vi "parce_string_to_elements.vi"(11 "BSONbytes":u8[](array[numeric]) format="%02x") -> (1 "restOfBytes":u8[](array[numeric]), 2 "sezeOK":bool, 3 "arrayOfElements":T1[](array[typedef]))   [LabVIEW 2015, in "BSON_convertors_Library.lvlib"]
doc: "Created by Artem Shevelev\nLabVIEW Portal profile: http://www.labviewportal.org/memberlist.php?mode=viewprofile&u=2340\ne-mail: artem.sh@gmail.com\nshevelev.pro"
uses:
  BSON_convertors_Library.lvlib
  typedefs/BSONelement.ctl
  typedefs/dataType.ctl
  typedefs/binaryData_cluster.ctl
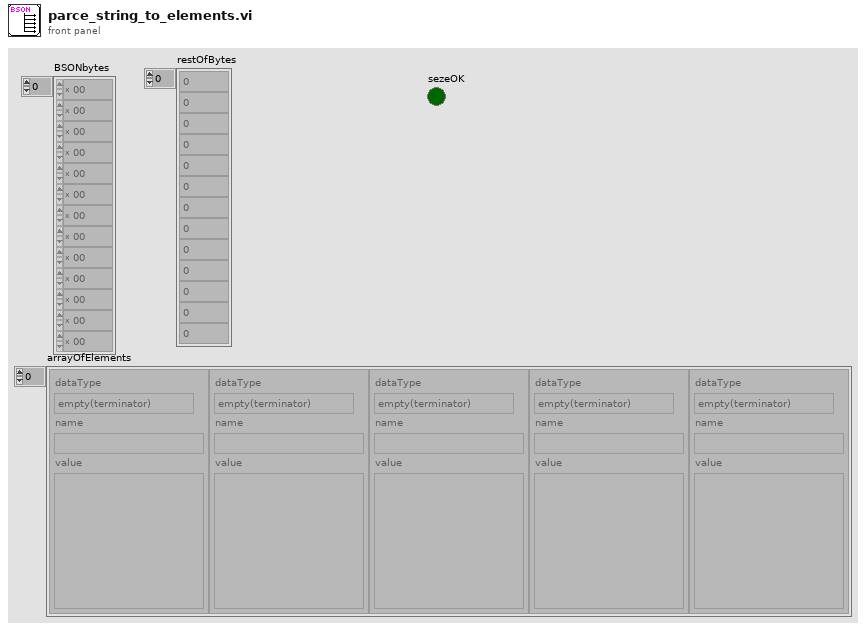
[diagram p1: front panel]
types:
  T1 = typedef "BSON_convertors_Library.lvlib/BSONelement.ctl" = cluster{"dataType":T2, "name":string, "value":variant}
  T2 = typedef "BSON_convertors_Library.lvlib/dataType.ctl" = enum8{"empty(terminator)", "double", "string", "document", "array", "binary", "Deprecated(Undefined)", "ObjectId", "boolean", "UTC datetime", "Null value", "cstring", "Deprecated(DBPointer)", "JavaScript", "Deprecated(Symbol)", "code_w_s", "int32", "uint64", "int64", "ext (decimal128)", "Min key", "Max key"}
  T3 = typedef "BSON_convertors_Library.lvlib/binaryData_cluster.ctl" = cluster{"subType":u8, "byteArray":u8[]}
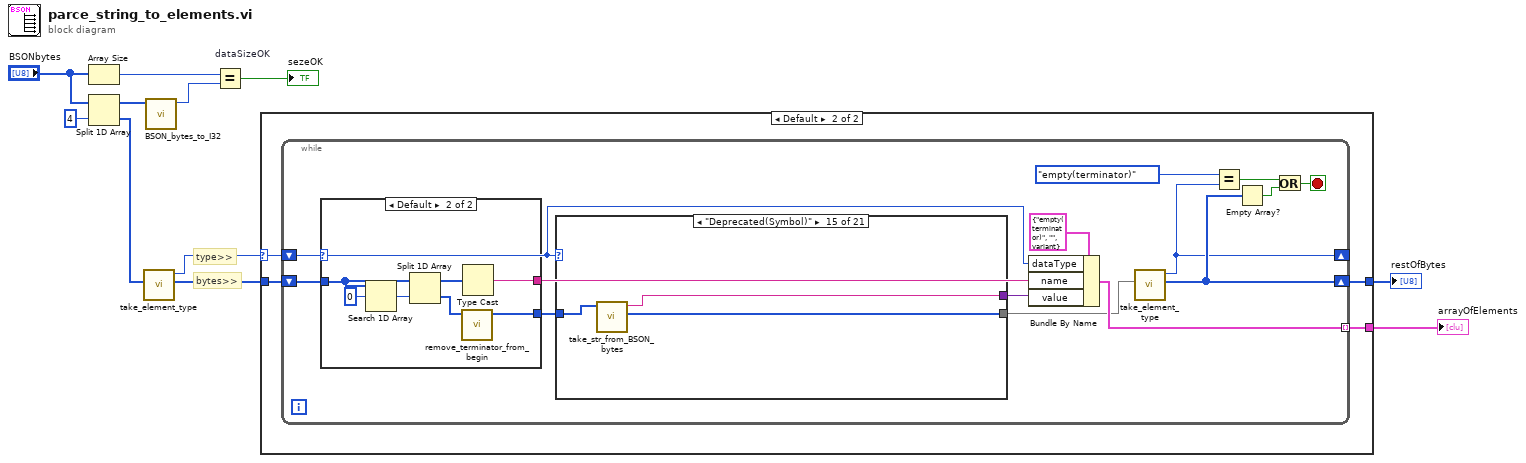
[diagram p0: block diagram]
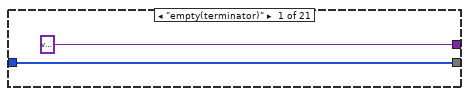
[diagram p4: hidden frame]
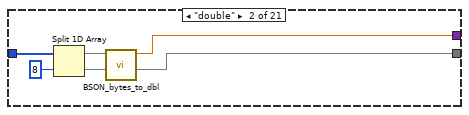
[diagram p5: hidden frame]
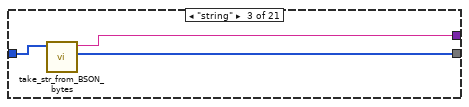
[diagram p6: hidden frame]
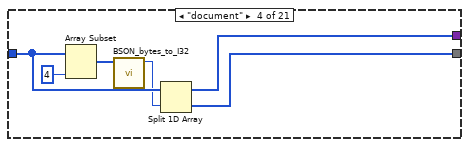
[diagram p7: hidden frame]
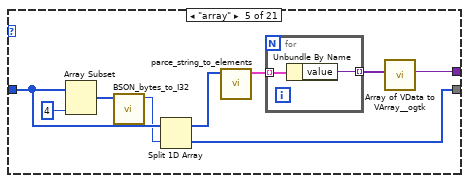
[diagram p8: hidden frame]
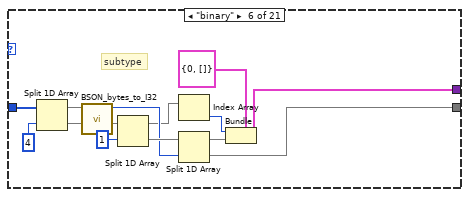
[diagram p9: hidden frame]
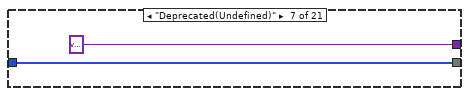
[diagram p10: hidden frame]
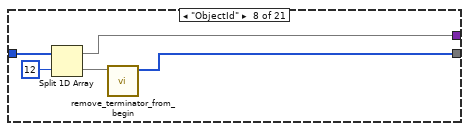
[diagram p11: hidden frame]
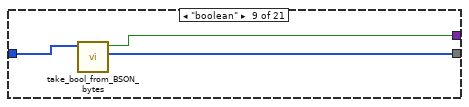
[diagram p12: hidden frame]
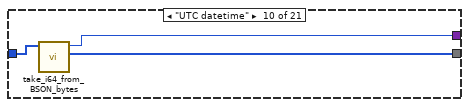
[diagram p13: hidden frame]
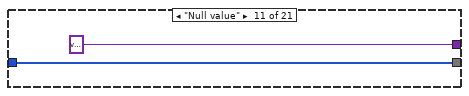
[diagram p14: hidden frame]
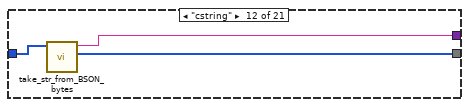
[diagram p15: hidden frame]
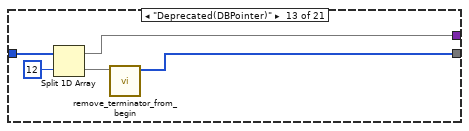
[diagram p16: hidden frame]
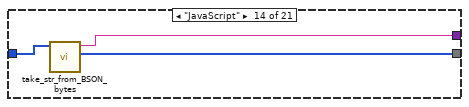
[diagram p17: hidden frame]
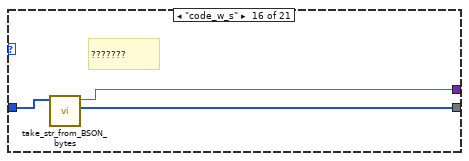
[diagram p18: hidden frame]
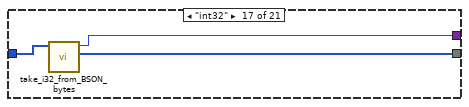
[diagram p19: hidden frame]
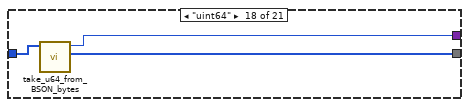
[diagram p20: hidden frame]
diagram:
  # "bytes>>"
  # "type>>"
  n1 = Array Size(array="BSONbytes") -> (size(s)=w8:i32)
  n2 = Split 1D Array(array="BSONbytes", index=4) -> (first subarray=w9:u8[], second subarray=w4:u8[])
  n3 = call "take_element_type.vi"("BSONbytes"=w4) -> ("restOfBytes"=w3:u8[], "dataType"=w2:T2)  [unwired: 9 in]
  n4 = call "BSON_bytes_to_I32.vi"("BSONbytes"=w9) -> ("value"=w7:i32)  [unwired: 10 in]
  n5 = Equal? "dataSizeOK"(x=w8, y=w7) -> (x = y?=→"sezeOK":bool)
  n6 = case shown="Default" w2 {
    selector: w2 -> [_ w14]
    tunnel: [_ w16] -> w5
    tunnel: w3 -> [w12 w15]
    tunnel: [w12 w13] -> w1
    frame "empty(terminator)" {
    }
    frame Default {
      n7 = while {
        shift-right: [w19] -> w13
        shift-left: w15 -> [w22]
        tunnel: [w24] -> w16 mode=indexing
        shift-right: [w17] -> _
        shift-left: w14 -> [w21]
        stop <- w25 stop-if-true
        n8 = case shown="Default" w21 {
          tunnel: w22 -> [w31 w37]
          tunnel: [_ w35] -> w29
          tunnel: [w31 w32] -> w23
          frame "empty(terminator)" {
            # "without name"
          }
          frame Default {
            n9 = Search 1D Array(1D array=w37, element=u8 0) -> (index of element=w36:i32)  [unwired: 1 in]
            n10 = Split 1D Array(array=w37, index=w36) -> (first subarray=w34:u8[], second subarray=w33:u8[])
            n11 = call "remove_terminator_from_begin.vi"("BSONbytes"=w33) -> ("restOfBytes"=w32:u8[])  [unwired: 10 in]
            n12 = Type Cast(x=w34) -> (*(type *) &x=w35:string)  [unwired: 1 in]
          }
        }
        n13 = case shown="\"Deprecated(Symbol)\"" w21 {
          tunnel: [variant w42 w47 w50 w55 w67 variant ("value") w83 w87 w90 variant ("value") w95 w99 w102 w105 w108 w112 w115 w118 w121 variant ("value")] -> w28
          tunnel: w23 -> [w39 w44 w48 w52 w61 w78 w80 w84 w88 w91 w93 w96 w100 w104 w107 w110 w113 w116 w119 w122 w124]
          tunnel: [w39 w41 w46 w49 w59 w68 w80 w81 w86 w89 w93 w94 w97 w103 w106 w109 w111 w114 w117 w120 w124] -> w20
          frame "empty(terminator)" {
          }
          frame "double" {
            n14 = Split 1D Array(array=w44, index=8) -> (first subarray=w43:u8[], second subarray=w41:u8[])
            n15 = call "BSON_bytes_to_dbl.vi"("BSONbytes"=w43) -> ("value"=w42:dbl)  [unwired: 10 in]
          }
          frame "string" {
            n16 = call "take_str_from_BSON_bytes.vi"("BSONbytes"=w48) -> ("restOfBytes"=w46:u8[], "value"=w47:string)  [unwired: 9 in]
          }
          frame "document" {
            n17 = Array Subset(array=w52, length=4 ("index")) -> (w54:u8[])  [unwired: 1 in]
            n18 = call "BSON_bytes_to_I32.vi"("BSONbytes"=w54) -> ("value"=w51:i32)  [unwired: 10 in]
            n19 = Split 1D Array(array=w52, index=w51) -> (first subarray=w50:u8[], second subarray=w49:u8[])
          }
          frame "array" {
            n20 = Array Subset(array=w61, length=4 ("index")) -> (w63:u8[])  [unwired: 1 in]
            n21 = call "BSON_bytes_to_I32.vi"("BSONbytes"=w63) -> ("value"=w60:i32)  [unwired: 10 in]
            n22 = Split 1D Array(array=w61, index=w60) -> (first subarray=w58:u8[], second subarray=w59:u8[])
            n23 = call "parce_string_to_elements.vi"("BSONbytes"=w58) -> ("arrayOfElements"=w57:T1[])  [unwired: 8 in, 2 out]
            n24 = for {
              tunnel: w57 -> [w65] mode=indexing
              tunnel: [w64] -> w56 mode=indexing
              n25 = Unbundle By Name(w65) -> ("value"=w64:variant)
            }
            n26 = call <userlib>:"Array of VData to VArray__ogtk.vi"("1D Array of VData"=w56) -> ("VArray"=w55:variant)  [unwired: 9 in, 1 out]
          }
          frame "binary" {
            # "subtype"
            n27 = Split 1D Array(array=w78, index=4) -> (first subarray=w76:u8[], second subarray=w75:u8[])
            n28 = call "BSON_bytes_to_I32.vi"("BSONbytes"=w76) -> ("value"=w72:i32)  [unwired: 10 in]
            n29 = Split 1D Array(array=w75, index=1) -> (first subarray=w71:u8[], second subarray=w73:u8[])
            n30 = Index Array(array=w71) -> (element=w70:u8)  [unwired: 1 in]
            n31 = Split 1D Array(array=w73, index=w72) -> (first subarray=w69:u8[], second subarray=w68:u8[])
            n32 = Bundle(cluster=T3 {"subType"=0, "byteArray"=[]}, "subType"=w70, "byteArray"=w69) -> (w67:T3)
          }
          frame "Deprecated(Undefined)" {
          }
          frame "ObjectId" {
            n33 = Split 1D Array(array=w84, index=12) -> (first subarray=w83:u8[], second subarray=w82:u8[])
            n34 = call "remove_terminator_from_begin.vi"("BSONbytes"=w82) -> ("restOfBytes"=w81:u8[])  [unwired: 10 in]
          }
          frame "boolean" {
            n35 = call "take_bool_from_BSON_bytes.vi"("BSONbytes"=w88) -> ("restOfBytes"=w86:u8[], "value"=w87:bool)  [unwired: 9 in]
          }
          frame "UTC datetime" {
            n36 = call "take_i64_from_BSON_bytes.vi"("BSONbytes"=w91) -> ("restOfBytes"=w89:u8[], "value"=w90:i64)  [unwired: 9 in]
          }
          frame "Null value" {
          }
          frame "cstring" {
            n37 = call "take_str_from_BSON_bytes.vi"("BSONbytes"=w96) -> ("restOfBytes"=w94:u8[], "value"=w95:string)  [unwired: 9 in]
          }
          frame "Deprecated(DBPointer)" {
            n38 = Split 1D Array(array=w100, index=12) -> (first subarray=w99:u8[], second subarray=w98:u8[])
            n39 = call "remove_terminator_from_begin.vi"("BSONbytes"=w98) -> ("restOfBytes"=w97:u8[])  [unwired: 10 in]
          }
          frame "JavaScript" {
            n40 = call "take_str_from_BSON_bytes.vi"("BSONbytes"=w104) -> ("restOfBytes"=w103:u8[], "value"=w102:string)  [unwired: 9 in]
          }
          frame "Deprecated(Symbol)" {
            n41 = call "take_str_from_BSON_bytes.vi"("BSONbytes"=w107) -> ("restOfBytes"=w106:u8[], "value"=w105:string)  [unwired: 9 in]
          }
          frame "code_w_s" {
            # "???????"
            n42 = call "take_str_from_BSON_bytes.vi"("BSONbytes"=w110) -> ("restOfBytes"=w109:u8[], "value"=w108:string)  [unwired: 9 in]
          }
          frame "int32" {
            n43 = call "take_i32_from_BSON_bytes.vi"("BSONbytes"=w113) -> ("restOfBytes"=w111:u8[], "value"=w112:i32)  [unwired: 9 in]
          }
          frame "uint64" {
            n44 = call "take_u64_from_BSON_bytes.vi"("BSONbytes"=w116) -> ("restOfBytes"=w114:u8[], "value"=w115:u64)  [unwired: 9 in]
          }
          frame "int64" {
            n45 = call "take_i64_from_BSON_bytes.vi"("BSONbytes"=w119) -> ("restOfBytes"=w117:u8[], "value"=w118:i64)  [unwired: 9 in]
          }
          frame "ext (decimal128)" {
            n46 = call "take_ext_from_BSON_bytes.vi"("BSONbytes"=w122) -> ("restOfBytes"=w120:u8[], "value"=w121:ext)  [unwired: 9 in]
          }
          frame "Min key", "Max key" {
            # "?????"
          }
        }
        n47 = Bundle By Name(cluster=T1 {"dataType"=enum."empty(terminator)", "name"="", "value"=variant} ("element"), "dataType"=w21, "name"=w29, "value"=w28) -> (w24:T1)
        n48 = call "take_element_type.vi"("BSONbytes"=w20) -> ("restOfBytes"=w19:u8[], "dataType"=w17:T2)  [unwired: 9 in]
        n49 = Equal?(x=dataType."empty(terminator)", y=w17) -> (x = y?=w26:bool)
        n50 = Empty Array?(array=w19) -> (empty?=w27:bool)
        n51 = Or(x=w26, y=w27) -> (x .or. y?=w25:bool)
      }
    }
  }
  "restOfBytes" <- w1
  "arrayOfElements" <- w5
